vi "Unflatten DBL.vi"(11 "Tag value":string) -> (3 "Numeric":dbl)   [LabVIEW 2020, in "NI_VIAn_XML Parsing.lvlib"]
uses:
  <vilib>/addons/analyzer/XML Parsing/NI_VIAn_XML Parsing.lvlib
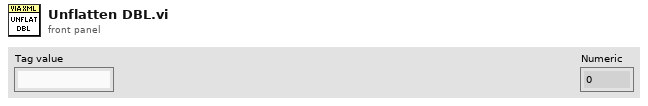
[diagram p1: front panel]
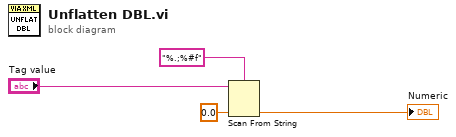
[diagram p0: block diagram]
diagram:
  n1 = Scan From String(format string="%.;%#f" ("initial string"), input string="Tag value", default 1=0.0 ("default value 1")) -> (output 1=→"Numeric":dbl)  [unwired: 2 in, 3 out]
